vi "Unflat JSON.vi"(8 "error in (no error)":errorcluster, 10 "JSON string":string, 11 "JSON reader in":refnum<class "JSON reader.lvclass">) -> (0 "error out":errorcluster, 3 "JSON reader out":refnum<class "JSON reader.lvclass">)   [LabVIEW 2018, in "JSON reader.lvclass"]
uses:
  JSON reader.lvclass
  Interface/Interface.lvclass
panel:
  out "CCD Config":T1
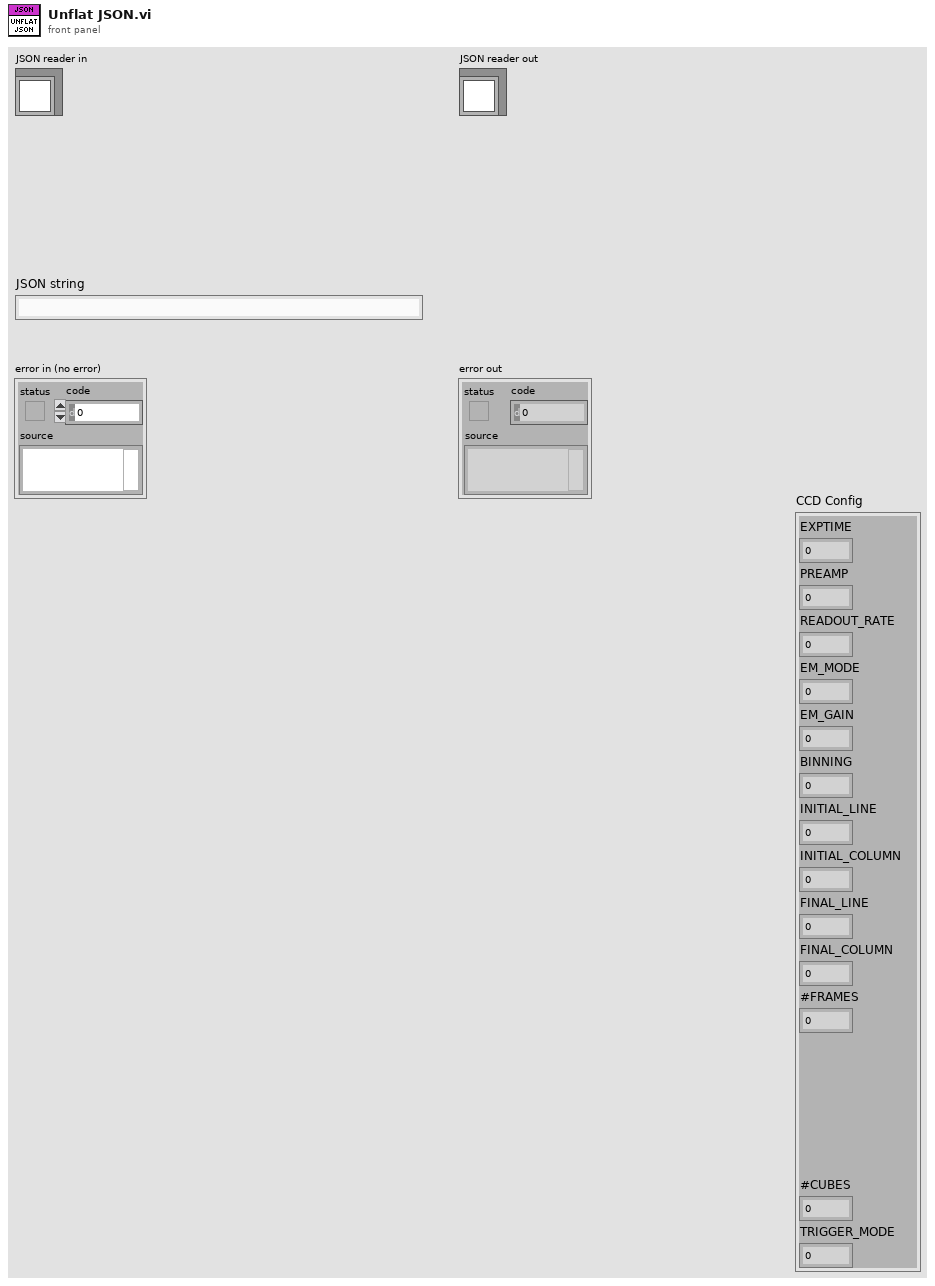
[diagram p1: front panel]
types:
  T1 = cluster{"EXPTIME":sgl, "PREAMP":u8, "READOUT_RATE":u8, "EM_MODE":u8, "EM_GAIN":u16, "BINNING":u16, "INITIAL_LINE":u16, "INITIAL_COLUMN":u16, "FINAL_LINE":u16, "FINAL_COLUMN":u16, "#FRAMES":u32, "#CUBES":u32, "TRIGGER_MODE":u16}
  T2 = cluster{"ACQUISITION_MODE":u8, "TRIGGER_MODE":u8, "READ_MODE":u8, "PREAMP":u8, "READOUT_RATE":u8, "VERTICAL_SHIFT_SPEED":u8, "EM_MODE":u8, "EM_GAIN":u16, "SHUTTER_MODE":u8, "SHUTTER_TTL":u8, "SHUTTER_OPENING_TIME":u16, "SHUTTER_CLOSING_TIME":u16, "VBIN":u16, "HBIN":u16, "INITIAL_LINE":u16, "INITIAL_COLUMN":u16, "FINAL_LINE":u16, "FINAL_COLUMN":u16, "FRAME_TRANSFER":bool, "VERTICAL_CLOCK_VOLTAGE":u8, "AD_CHANNEL":u32}
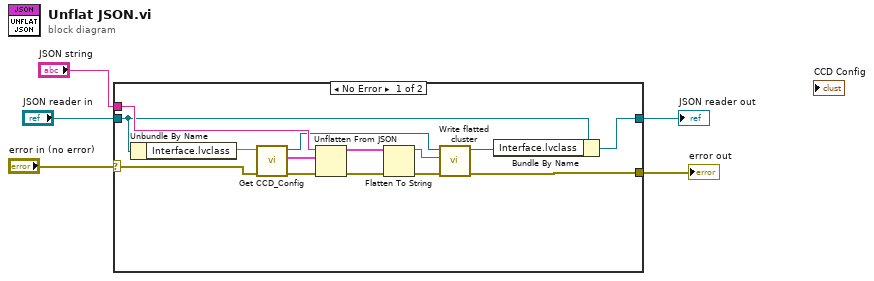
[diagram p0: block diagram]
diagram:
  n1 = case shown="No Error" "error in (no error)" {
    selector: "error in (no error)" -> [w17 w21]
    tunnel: [w9 w21] -> w4
    tunnel: [w6 w20] -> w2
    tunnel: "JSON reader in" -> [w8 w20]
    tunnel: "JSON string" -> [w19 _]
    frame No Error {
      n2 = Unbundle By Name(w8) -> ("Interface.lvclass"=w18)
      n3 = call-dynamic "Get CCD_Config.vi"("error in (no error)"=w17, "Interface in"=w18) -> ("error out"=w16:errorcluster, "output cluster"=w15:T2, "Interface out"=w14:refnum<class "Interface.lvclass">)  [unwired: 7 in]
      n4 = Unflatten From JSON(JSON string=w19, type and defaults=w15, error in (no error)=w16) -> (value=w12:T2, error out=w13:errorcluster)  [unwired: 4 in]
      n5 = Flatten To String(anything=w12, error in (no error)=w13) -> (data string=w11:string, error out=w10:errorcluster)  [unwired: 2 in, 1 out]
      n6 = call "Write flatted cluster.vi"("error in (no error)"=w10, "flatted cluster"=w11, "Interface in"=w14) -> ("error out"=w9:errorcluster, "Interface out"=w7:refnum<class "Interface.lvclass">)  [unwired: 7 in]
      n7 = Bundle By Name(cluster=w8, "Interface.lvclass"=w7) -> (w6:refnum<class "JSON reader.lvclass">)
    }
    frame Error {
    }
  }
  "error out" <- w4
  "JSON reader out" <- w2
